vi "GetTimingSession.vi"(8 "error in (no error)":errorcluster, 11 "PXI_MultiTrig in":refnum<class "PXI_MultiTrig.lvclass">) -> (0 "error out":errorcluster, 2 "TimingSession":variant, 3 "PXI_MultiTrig out":refnum<class "PXI_MultiTrig.lvclass">)   [LabVIEW 2018, in "SyncPlugins.lvlib" / "PXI_MultiTrig.lvclass"]
uses:
  PXI_MultiTrig.lvclass
  PXI_MultiTrig.lvclass/PXI_MultiTrig.ctl
  Accessors/Read RefClkSession.vi
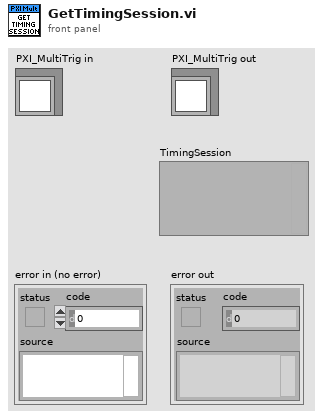
[diagram p1: front panel]
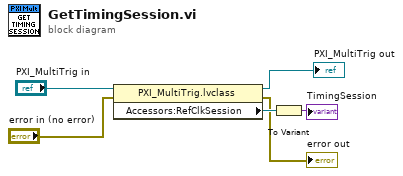
[diagram p0: block diagram]
diagram:
  n1 = property class="PXI_MultiTrig.lvclass"(reference="PXI_MultiTrig in", error in="error in (no error)") -> (reference out=→"PXI_MultiTrig out":refnum<class "PXI_MultiTrig.lvclass">, error out=→"error out":errorcluster, "Accessors:RefClkSession"=w4:refnum<k15>)
  n2 = To Variant(anything=w4) -> (Variant=→"TimingSession":variant)
